vi "send_LVCellValues.vi"(4 "Counter":i32, 5 "200/freq":i32=20, 6 "Active":bool, 7 "CAN ID":u32=1074 format="%x", 8 "Message":T2={"Voltage [mV]"=3968.3673469387754, "Temp [C°]"=31.836734693877553, "CELL ID"=0, "Discharge"=FALSE, "Volt error"=0, "Temp error"=0} {"Temp [C°]" scale=0.0..80.0; "Voltage [mV]" scale=3000.0..4300.0}, 11 "CAN frame":T1[](array[typedef]) {"Data" format="%.0x"; "ArbitrationId" format="%.0x"; "Timestamp" format="%<%I:%M:%S%3u %p\n%m/%d/%Y>T"}) -> (3 "CAN frame out":T1[](array[typedef]) {"Data" format="%.0x"; "ArbitrationId" format="%.0x"; "Timestamp" format="%<%I:%M:%S%3u %p\n%m/%d/%Y>T"})   [LabVIEW 2017]
uses:
  <vilib>/nican/nican.llb/CanFrameTimed.ctl
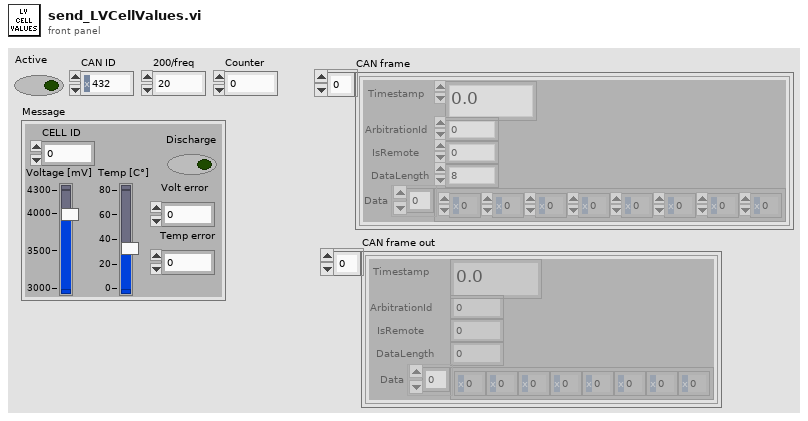
[diagram p1: front panel]
types:
  T1 = typedef "CanFrameTimed.ctl" = cluster{"Timestamp":dbl, "ArbitrationId":u32, "IsRemote":u8, "DataLength":u8, "Data":u8[]}
  T2 = cluster{"Voltage [mV]":dbl, "Temp [C°]":dbl, "CELL ID":u8, "Discharge":bool, "Volt error":u8, "Temp error":u8}
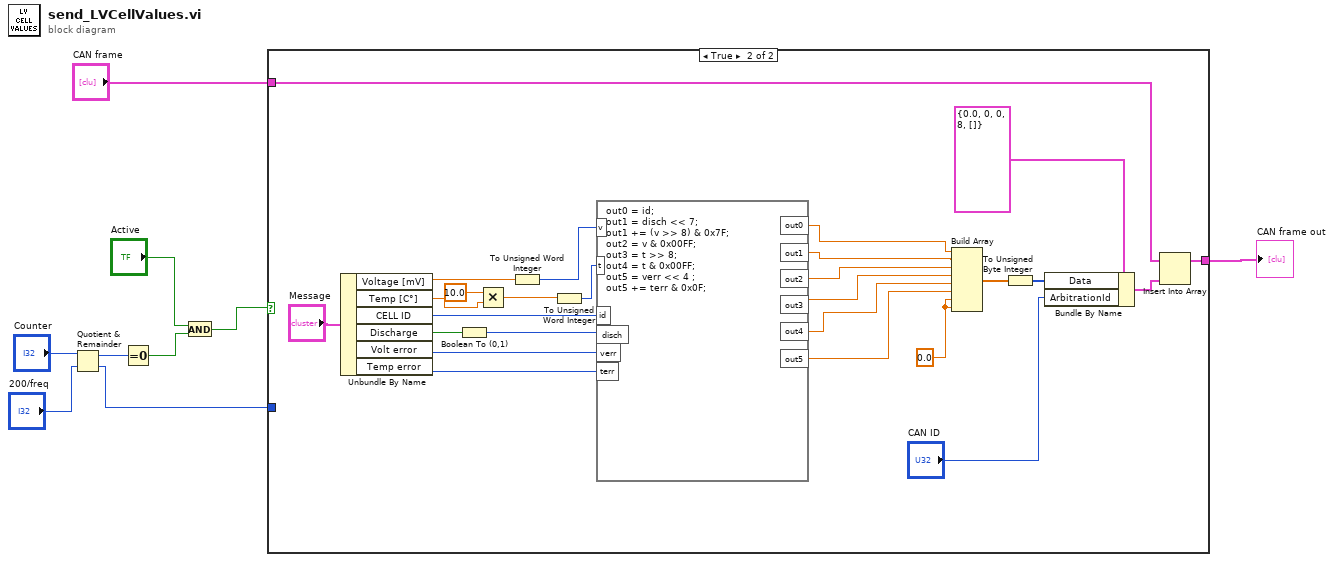
[diagram p0: block diagram]
diagram:
  n1 = Quotient & Remainder(x="Counter", y="200/freq") -> (x-y*floor(x/y)=w6:i32, floor(x/y)=w1:i32)
  n2 = Equal To 0?(x=w6) -> (x = 0?=w4:bool)
  n3 = And(x="Active", y=w4) -> (x .and. y?=w3:bool)
  n4 = case shown="True" w3 {
    tunnel: "CAN frame" -> [w10 w27]
    tunnel: [w10 w25] -> w8
    tunnel: w1 -> [_ _]
    frame False {
    }
    frame True {
      w22 = 0.0 ("element")
      n5 = Unbundle By Name("Message") -> ("Voltage [mV]"=w16:dbl, "Temp [C°]"=w20:dbl, "CELL ID"=w17:u8, "Discharge"=w14:bool, "Volt error"=w12:u8, "Temp error"=w11:u8)
      n6 = Boolean To (0,1)(Boolean=w14) -> (0, 1=w13:i16)
      n7 = Multiply(x=10.0, y=w20) -> (x*y=w19:dbl)
      n8 = To Unsigned Word Integer(number=w16) -> (unsigned 16bit integer=w23:u16)
      n9 = To Unsigned Word Integer(number=w19) -> (unsigned 16bit integer=w36:u16)
      n10 = formula code="out0 = id;\nout1 = disch << 7;\nout1 += (v >> 8) & 0x7F;\nout2 = v & 0x00FF;\nout3 = t >> 8;\nout4 = t & 0x00FF;\nout5 = verr << 4 ;\nout5 += terr & 0x0F;"("t"=w36, "v"=w23, "id"=w17, "disch"=w13, "verr"=w12, "terr"=w11) -> ("out1"=w34:dbl, "out2"=w33:dbl, "out3"=w32:dbl, "out0"=w35:dbl, "out4"=w31:dbl, "out5"=w15:dbl)
      n11 = Build Array(w35, w34, w33, w32, w31, w15, w22, w22) -> (w30:dbl[])
      n12 = To Unsigned Byte Integer(number=w30) -> (unsigned 8bit integer=w29:u8[])
      n13 = Bundle By Name(cluster=T1 {"Timestamp"=0.0, "ArbitrationId"=0, "IsRemote"=0, "DataLength"=8, "Data"=[]} ("CAN frame"), "Data"=w29, "ArbitrationId"="CAN ID") -> (w26:T1)
      n14 = Insert Into Array(array=w27, new element=w26) -> (w25:T1[])  [unwired: 1 in]
    }
  }
  "CAN frame out" <- w8
